vi "RSZVB Select More Ratios Generator.vi"(0 "VISA session":refnum<visa-resource-name>, 1 "Numerator Type (a)":i32(ring) items=["a", "b"], 2 "Denominator Type (a)":i32(ring) items=["a", "b"], 5 "Channel (1)":i32=1, 7 "Trace Name (\"Trc1\")":string="Trc1", 9 "Generator Number (1)":i32=1, 11 "error in (no error)":errorcluster {"code" format="%.0x"}, 12 "Numerator Port Number (1)":i32=1, 13 "Denominator Port Number (1)":i32=1) -> (4 "dup VISA session":refnum<visa-resource-name>, 15 "error out":errorcluster {"code" format="%.0x"})   [LabVIEW 2011]
doc: "This VI select arbitrary ratios of wave quantities, e.g. for different detectors and external generator.\n\nAssigns a measurement parameter to an existing trace or creates a trace and assigns a channel number, a name and a measurement parameter to it. The trace is not displayed.\n\nThe notation for ratios and the functionality of the More Ratios dialog is analogous to the definition of S-parameters.\n\nRatio of wave quantities with port numbers and external generator providing the stimulus signal.\n\nRemote-control command(s):\nCALCulate<Ch>:PARameter:SDEFine '<string>', 'B2G1/A1G1' | 'B1G1/A1G1' | 'B2G1/B1G1' | 'B1G1/B2G1' | ...\nCALCulate<Ch>:PARameter:MEASure '<string>', 'B2G1/A1G1' | 'B1G1/A1G1' | 'B2G1/B1G1' | 'B1G1/B2G1' | ..."
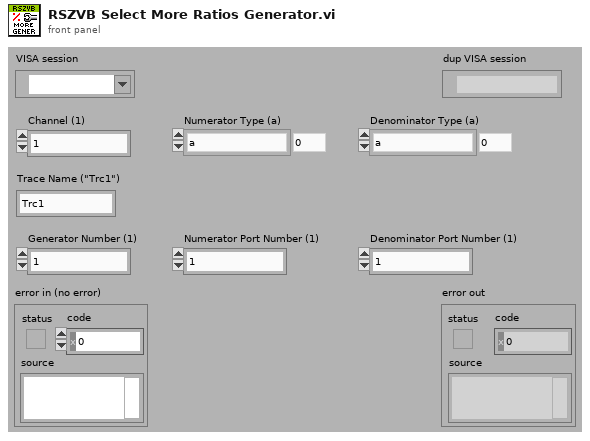
[diagram p1: front panel]
types:
  T1 = cluster{"Error Checking (T: On)":bool, "Installed Options":string[], "Data Valid?":bool, "Ports":i32, "Model":string[], "Option Checking (T: On)":bool}
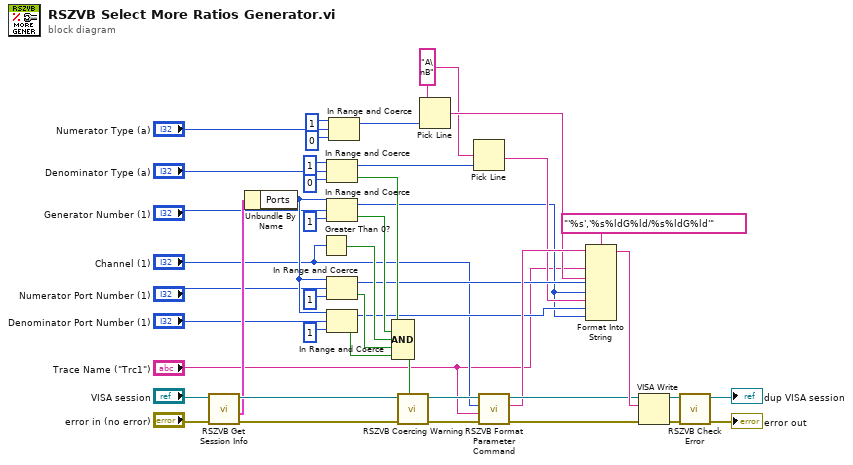
[diagram p0: block diagram]
diagram:
  w19 = "A\nB"
  n1 = call "RSZVB Get Session Info.vi"("error in (no error)"="error in (no error)", "VISA session"="VISA session") -> ("error out"=w15:errorcluster, "Session Info"=w13:T1, "dup VISA session"=w14:refnum<visa-resource-name>)  [unwired: 7 in]
  n2 = Unbundle By Name(w13) -> ("Ports"=w12:i32)
  n3 = Greater Than 0?(x="Channel (1)") -> (x > 0?=w27:bool)
  n4 = In Range and Coerce(upper limit=1, x="Denominator Type (a)", lower limit=0) -> (coerced(x)=w30:i32, In Range?=w29:bool)
  n5 = In Range and Coerce(upper limit=w12, x="Generator Number (1)", lower limit=1) -> (coerced(x)=w16:i32, In Range?=w28:bool)
  n6 = In Range and Coerce(upper limit=w12, x="Numerator Port Number (1)", lower limit=1) -> (coerced(x)=w21:i32, In Range?=w26:bool)
  n7 = In Range and Coerce(upper limit=w12, x="Denominator Port Number (1)", lower limit=1) -> (coerced(x)=w18:i32, In Range?=w25:bool)
  n8 = In Range and Coerce(upper limit=1, x="Numerator Type (a)", lower limit=0) -> (coerced(x)=w22:i32)  [unwired: 1 out]
  n9 = Compound Arithmetic op=AND(w29, w28, w27, w26, w25) -> (w41:bool)
  n10 = call "RSZVB Coercing Warning.vi"("In Range?"=w41, "error in (no error)"=w15, "VISA session"=w14) -> ("error out"=w38:errorcluster, "dup VISA session"=w37:refnum<visa-resource-name>)  [unwired: 7 in]
  n11 = Pick Line(multi-line string=w19, line index=w22) -> (output string=w20:string)  [unwired: 1 in]
  n12 = Pick Line(multi-line string=w19, line index=w30) -> (output string=w17:string)  [unwired: 1 in]
  n13 = call "RSZVB Format Parameter Command.vi"("error in (no error)"=w38, "Trace Name (Trc1)"="Trace Name (\"Trc1\")", "Channel (1)"="Channel (1)", "VISA session"=w37) -> ("error out"=w39:errorcluster, "Buffer"=w34:string, "dup VISA session"=w36:refnum<visa-resource-name>)  [unwired: 5 in]
  n14 = Format Into String(format string="'%s','%s%ldG%ld/%s%ldG%ld'", initial string=w34, "Trace Name (\"Trc1\")", w20, w21, w16, w17, w18, w16) -> (resulting string=w40:string)  [unwired: 1 in, 1 out]
  n15 = VISA Write(VISA resource name=w36, write buffer=w40, error in (no error)=w39) -> (VISA resource name out=w42:refnum<visa-resource-name>, error out=w43:errorcluster)  [unwired: 1 out]
  n16 = call "RSZVB Check Error.vi"("error in (no error)"=w43, "VISA session"=w42) -> ("error out"=→"error out":errorcluster, "dup VISA session"=→"dup VISA session":refnum<visa-resource-name>)  [unwired: 8 in]
